vi "Get Configured Status Channels.vi"(8 "error in (no error)":errorcluster, 11 "VeriStand Data Sharing Framework in":refnum<class "VeriStand DSF.lvclass">) -> (0 "error out":errorcluster, 1 "status channels refs":T1[](array[typedef]) format="%.0x", 2 "status channel offsets":u64[](array[numeric]) format="%.0x", 3 "VeriStand Data Sharing Framework out":refnum<class "VeriStand DSF.lvclass">)   [LabVIEW 2017, in "DSF Engine.lvlib" / "VeriStand DSF.lvclass"]
uses:
  VeriStand DSF.lvclass
  <vilib>/NI Veristand/Custom Device API/Custom Device Item Ref.ctl
  VeriStand DSF.lvclass/VeriStand DSF.ctl
  <vilib>/NI Veristand/Custom Device API/Data Access Type.ctl
  <vilib>/NI Veristand/Custom Device API/Custom Device API.lvlib
  Shared/DSF Shared.lvlib
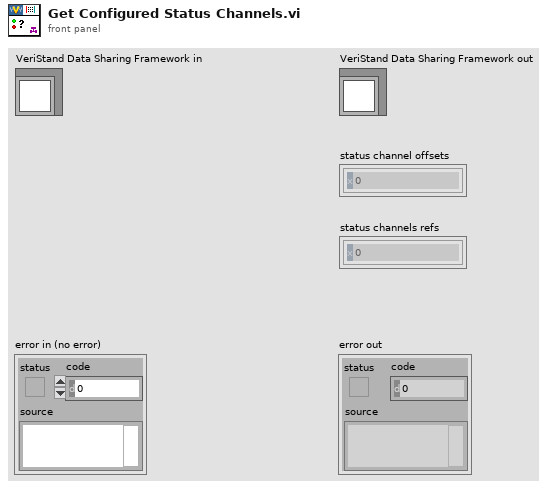
[diagram p1: front panel]
types:
  T1 = typedef "Custom Device API.lvlib/Custom Device Item Ref.ctl" = u64
  T2 = typedef "Custom Device API.lvlib/Data Access Type.ctl" = enum16{"Read", "Write"}
  T3 = typedef "Custom Device API.lvlib/Data Reference.ctl" = i32
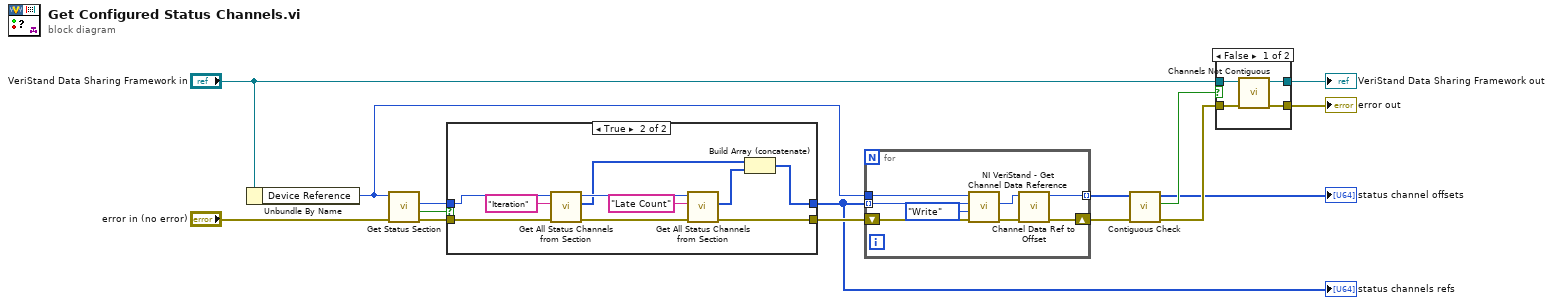
[diagram p0: block diagram]
diagram:
  n1 = Unbundle By Name("VeriStand Data Sharing Framework in") -> ("Device Reference"=w9:T1)
  n2 = call "Get Status Section.vi"("error in (no error)"="error in (no error)", "Item Ref in"=w9) -> ("error out"=w14:errorcluster, "found"=w3:bool, "Status Section ref"=w13:T1)  [unwired: 6 in, 1 out]
  n3 = case shown="True" w3 {
    tunnel: w14 -> [w16 w25]
    tunnel: w13 -> [_ w24]
    tunnel: [w16 w17] -> w12
    tunnel: [_ w26] -> w2
    frame False {
    }
    frame True {
      n4 = call "Get All Status Channels from Section.vi"("error in (no error)"=w25, "Section Name"="Iteration", "Item Ref in"=w24) -> ("error out"=w21:errorcluster, "status channels refs"=w19:T1[], "Item Ref out"=w22:T1)  [unwired: 6 in]
      n5 = call "Get All Status Channels from Section.vi"("error in (no error)"=w21, "Section Name"="Late Count", "Item Ref in"=w22) -> ("error out"=w17:errorcluster, "status channels refs"=w18:T1[])  [unwired: 6 in, 1 out]
      n6 = Build Array (concatenate)(w19, w18) -> (w26:T1[])
    }
  }
  "status channels refs" <- w2
  n7 = for {
    shift-right: [w33] -> w11
    shift-left: w12 -> [w32]
    tunnel: [w30] -> w10 mode=indexing
    tunnel: w9 -> [w28]
    tunnel: w2 -> [w27] mode=indexing
    n8 = call <vilib>:"NI VeriStand - Get Channel Data Reference.vi"("error in (no error)"=w32, "Access"=Data_Access_Type."Write", "Channel Ref in"=w27, "Device Ref in"=w28) -> ("error out"=w34:errorcluster, "Channel Data Reference"=w31:T3)  [unwired: 5 in, 1 out]
    n9 = call "Channel Data Ref to Offset.vi"("error in (no error)"=w34, "Channel Data Reference"=w31) -> ("error out"=w33:errorcluster, "channel offset"=w30:u64)  [unwired: 8 in]
  }
  n10 = call "Contiguous Check.vi"("error in (no error)"=w11, "channel offsets in"=w10) -> ("error out"=w5:errorcluster, "contiguous?"=w4:bool, "channel offsets out"=→"status channel offsets":u64[])  [unwired: 7 in]
  n11 = case shown="False" w4 {
    tunnel: "VeriStand Data Sharing Framework in" -> [w38 w40]
    tunnel: [w37 w40] -> w7
    tunnel: [w36 w39] -> w6
    tunnel: w5 -> [w35 w39]
    frame False {
      n12 = call "Channels Not Contiguous.vi"("error in (no error)"=w35, "VeriStand DSF in"=w38) -> ("error out"=w36:errorcluster, "VeriStand DSF out"=w37:refnum<class "VeriStand DSF.lvclass">)  [unwired: 8 in]
    }
    frame True {
    }
  }
  "error out" <- w6
  "VeriStand Data Sharing Framework out" <- w7
